vi "MaskfromArray.vi"(9 "cols":i32, 10 "rows":i32, 11 "Array":dbl[][](array[numeric])) -> (3 "Image Pixels (U8)":u8[][](array[numeric]))   [LabVIEW 2015]
uses:
  <vilib>/vision/NI_Vision_Development_Module.lvlib
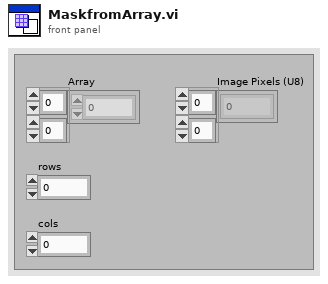
[diagram p1: front panel]
types:
  T1 = typedef "Image Type" = u32
  T2 = typedef "IMAQ Image.ctl" = refnum<image>
  T3 = typedef "ROI Descriptor" = cluster{"Global Rectangle":i32[], "Contours":cluster{"ID":enum32{"External", "Internal"}, "Type":u32, "Coordinates":i32[]}[]}
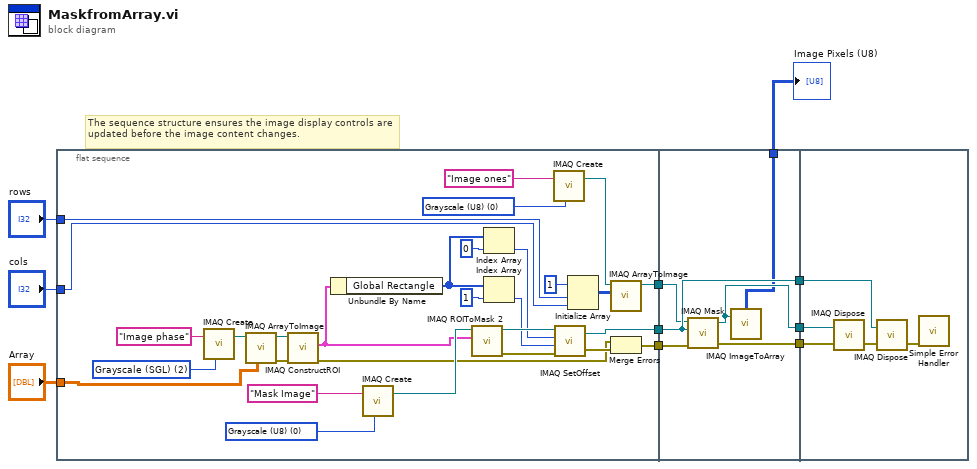
[diagram p0: block diagram]
diagram:
  # "The sequence structure ensures the image display controls are updated before the image content changes."
  n1 = flat-sequence {
    tunnel: [w36] -> w10
    tunnel: [w35] -> w9
    tunnel: "rows" -> [w18]
    tunnel: [w26] -> w8
    tunnel: "Array" -> [w23]
    tunnel: "cols" -> [w17]
    tunnel: [w41] -> w7
    tunnel: [w45] -> w6
    tunnel: [w44] -> w5
    tunnel: w10 -> [w44]
    tunnel: w9 -> [w43]
    tunnel: w8 -> [w42]
    tunnel: [w40] -> w4
    tunnel: w7 -> [w48]
    tunnel: w6 -> [w47]
    tunnel: w5 -> [w46]
    frame #0 {
      w24 = T1 2 items=["Grayscale (U8)", "Grayscale (I16)", "Grayscale (SGL)", "Complex (CSG)", "RGB (U32)", "HSL (U32)", "RGB (U64)", "Grayscale (U16)"] ("Image Type")
      w27 = T1 0 items=["Grayscale (U8)", "Grayscale (I16)", "Grayscale (SGL)", "Complex (CSG)", "RGB (U32)", "HSL (U32)", "RGB (U64)", "Grayscale (U16)"] ("Image Type")
      w38 = T1 0 items=["Grayscale (U8)", "Grayscale (I16)", "Grayscale (SGL)", "Complex (CSG)", "RGB (U32)", "HSL (U32)", "RGB (U64)", "Grayscale (U16)"] ("Image Type")
      n2 = call "IMAQ Create"("Image Name"="Image phase", "Image Type"=w24) -> ("New Image"=w25:T2)  [unwired: 3 in, 1 out]
      n3 = call "IMAQ ArrayToImage"("Image Pixels (Float)"=w23, "Image"=w25) -> ("error out"=w21:errorcluster, "Image Out"=w20:T2)  [unwired: 8 in]
      n4 = call "IMAQ ConstructROI"("error in (no error)"=w21, "Image"=w20) -> ("error out"=w19:errorcluster, "ROI Descriptor Out"=w16:T3)  [unwired: 6 in, 2 out]
      n5 = Unbundle By Name(w16) -> ("Global Rectangle"=w13:i32[])
      n6 = call "IMAQ Create"("Image Name"="Mask Image", "Image Type"=w38) -> ("New Image"=w34:T2)  [unwired: 3 in, 1 out]
      n7 = call "IMAQ ROIToMask 2"("ROI Descriptor"=w16, "Image"=w34) -> ("error out"=w32:errorcluster, "Image Out"=w33:T2)  [unwired: 7 in, 1 out]
      n8 = Index Array(array=w13, index=0) -> (element=w14:i32)
      n9 = Index Array(array=w13, index=1) -> (element=w11:i32)
      n10 = call "IMAQ Create"("Image Name"="Image ones", "Image Type"=w27) -> ("New Image"=w28:T2)  [unwired: 3 in, 1 out]
      n11 = call "IMAQ SetOffset"("error in (no error)"=w32, "Y Offset"=w11, "X Offset"=w14, "Image"=w33) -> ("error out"=w37:errorcluster, "Image Out"=w36:T2)
      n12 = Initialize Array(1, w18, w17) -> (w30:i32[][])
      n13 = call "IMAQ ArrayToImage"("Image Pixels (U8)"=w30, "Image"=w28) -> ("Image Out"=w26:T2)  [unwired: 8 in, 1 out]
      n14 = Merge Errors(w19, w37) -> (w35:errorcluster)
    }
    frame #1 {
      n15 = call "IMAQ Mask"("error in (no error)"=w43, "Image Mask"=w44, "Image Src"=w42) -> ("error out"=w45:errorcluster, "Image Dst Out"=w41:T2)  [unwired: 2 in]
      n16 = call "IMAQ ImageToArray"("Image"=w41) -> ("Image Pixels (U8)"=w40:u8[][])  [unwired: 3 in, 4 out]
    }
    frame #2 {
      n17 = call "IMAQ Dispose"("Image"=w48, "error in (no error)"=w47) -> ("error out"=w49:errorcluster)  [unwired: 4 in]
      n18 = call "IMAQ Dispose"("Image"=w46, "error in (no error)"=w49) -> ("error out"=w50:errorcluster)  [unwired: 4 in]
      n19 = call <vilib>:"Simple Error Handler.vi"("error in (no error)"=w50) -> ()  [unwired: 4 in, 5 out]
    }
  }
  "Image Pixels (U8)" <- w4
